vi "practica10RNA.vi"() -> ()   [LabVIEW 2016]
panel:
  in  "w2":dbl
  in  "w1":dbl
  in  "X2":dbl
  in  "X1":dbl
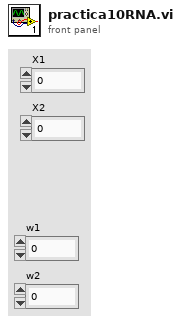
[diagram p1: front panel]
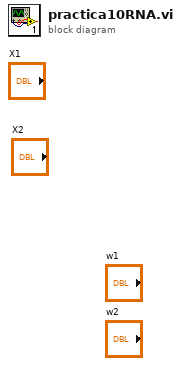
[diagram p0: block diagram]
diagram:
